vi "Untitled 4.vi"() -> ()   [LabVIEW 2020]
uses:
  Libraries/HslCommunication/Inovance5UTcp/Inovance5UTcp.lvclass
panel:
  out "Image":T1(plugin-control)
  out "data":bool
  in  "ipAddress":string
  in  "station":u8
  in  "port":i32
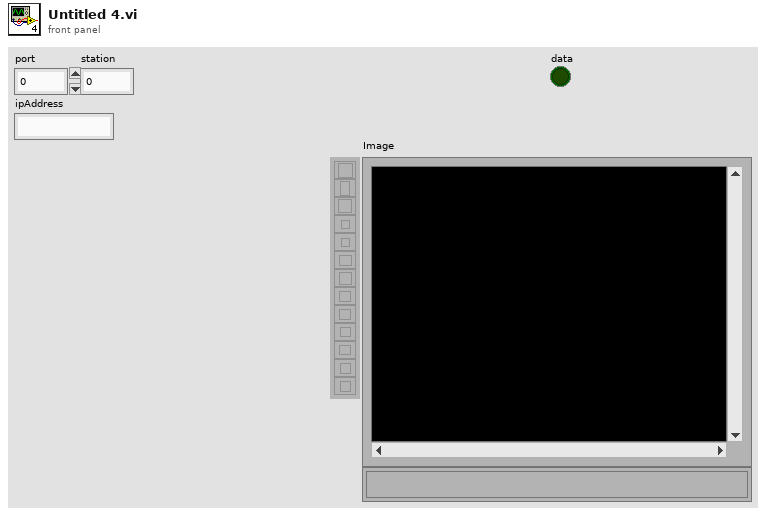
[diagram p1: front panel]
types:
  T1 = typedef "IMAQ Image.ctl" = refnum<image>
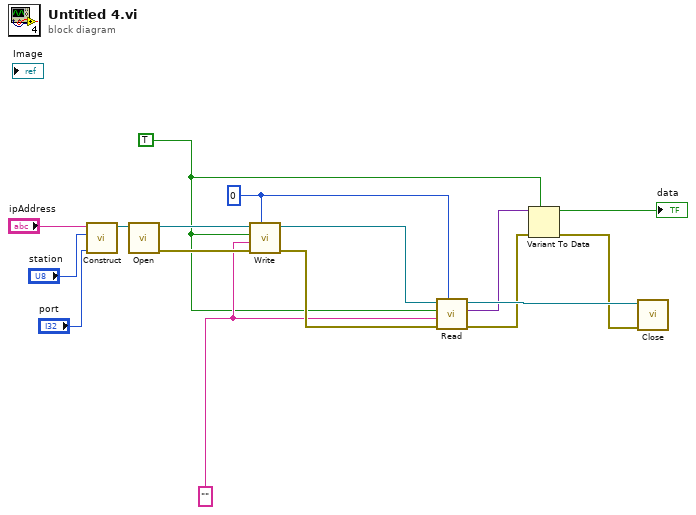
[diagram p0: block diagram]
diagram:
  w6 = u16 0 ("length")
  w7 = "" ("Start address")
  w4 = TRUE
  n1 = call "Construct.vi"("port"="port", "station"="station", "ipAddress"="ipAddress") -> ("MelsecMcNet out"=w16:refnum<class "Inovance5UTcp.lvclass">)  [unwired: 8 in]
  n2 = call-dynamic "Open.vi"("MelsecTCP in"=w16) -> ("error out"=w14:errorcluster, "MelsecTCP out"=w15:refnum<class "Inovance5UTcp.lvclass">)  [unwired: 8 in, 1 out]
  n3 = call "Write.vi"("length"=w6, "error in (no error)"=w14, "Start address"=w7, "Read Type"=w4, "MelsecTCP in"=w15) -> ("error out"=w9:errorcluster, "MelsecTCP out"=w10:refnum<class "Inovance5UTcp.lvclass">)  [unwired: 5 in]
  n4 = call "Read.vi"("length"=w6, "error in (no error)"=w9, "Start address"=w7, "Read Type"=w4, "MelsecTCP in"=w10) -> ("error out"=w3:errorcluster, "Data"=w5:variant, "MelsecTCP out"=w8:refnum<class "Inovance5UTcp.lvclass">)  [unwired: 4 in]
  n5 = Variant To Data(error in=w3, type=w4, Variant=w5) -> (data=→"data":bool, error out=w2:errorcluster)
  n6 = call-dynamic "Close.vi"("error in (no error)"=w2, "MelsecTCP in"=w8) -> ()  [unwired: 8 in, 2 out]
